vi "Test Move Vertically Outside World.vi"(8 "error in (no error)":errorcluster, 11 "Test Case In":refnum<class "World Test.lvclass">) -> (0 "error out":errorcluster, 3 "Test Case Out":refnum<class "World Test.lvclass">)   [LabVIEW 2020, in "World Test.lvclass"]
uses:
  World Test.lvclass
  C:/Program Files (x86)/National Instruments/LabVIEW 2020/vi.lib/Astemes/LUnit/Test Case.lvclass
  source/Particle/Position.ctl
  source/Particle.lvclass/Particle.ctl
  <vilib>/Astemes/LUnit/Test Case.lvclass/Test Case.ctl
  01074fa8-ee8a-411d-bc8b-fc92c4f90959.vi
  <vilib>/Astemes/LUnit/Palette/Pass.vi
  <vilib>/Astemes/LUnit/Palette/Fail.vi
  <vilib>/Astemes/LUnit/Compare Variants.vi
  <vilib>/Astemes/LUnit/Describe Comparison.vi
  <vilib>/Astemes/LUnit/Set Assertion Type.vi
  <vilib>/Astemes/LUnit/Add test result.vi
  <vilib>/Astemes/LUnit/Variant to string.vi
  <vilib>/Astemes/LUnit/LUnit Record Assertion Result.vi
  <vilib>/Astemes/LUnit/LUnit Aggregate Assertion Results.vi
  <vilib>/Astemes/LUnit/Method Result/LUnit Merge Status.vi
  <vilib>/Astemes/LUnit/LUnit Concatenate result strings.vi
  <vilib>/Utility/Data Type/Get Type Information.vi
  <vilib>/Utility/LVClass/Get LV Class Name.vi
  World Test.lvclass/World Test.ctl
  source/World/World.lvclass
  source/Particle.lvclass
panel:
  out "Position":T1
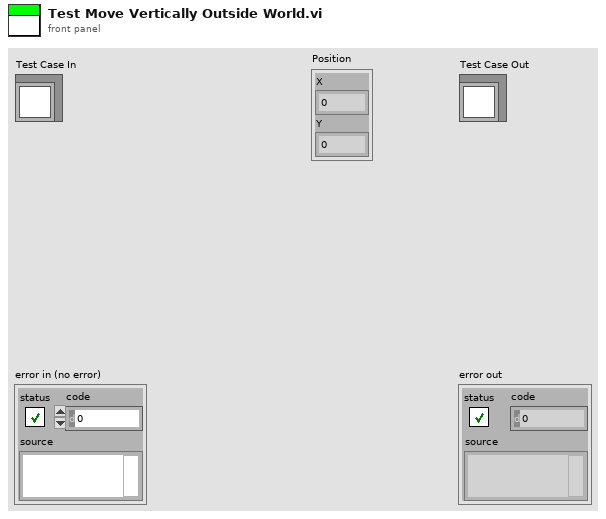
[diagram p1: front panel]
types:
  T1 = typedef "Particle.lvclass/Position.ctl" = cluster{"X":i32, "Y":i32}
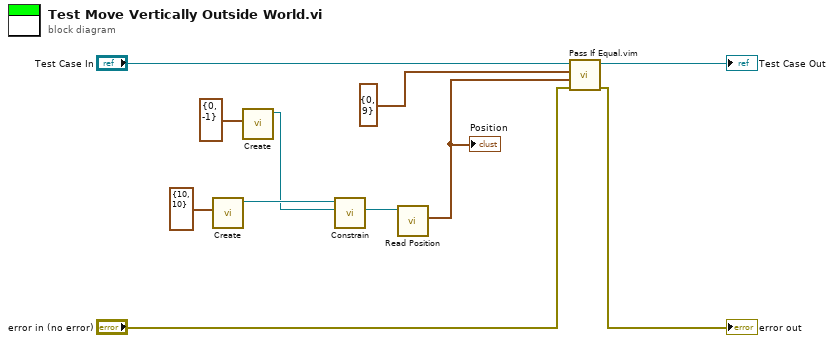
[diagram p0: block diagram]
diagram:
  n1 = call "Create.vi"("Size"=T1 {"X"=10, "Y"=10}) -> ("World out"=w5:refnum<class "World.lvclass">)  [unwired: 10 in]
  n2 = call "Create.vi"("Position"=T1 {"X"=0, "Y"=-1}) -> ("Particle out"=w4:refnum<class "Particle.lvclass">)  [unwired: 10 in]
  n3 = call "Constrain.vi"("Particle.lvclass"=w4, "World in"=w5) -> ("Particle"=w3:refnum<class "Particle.lvclass">)  [unwired: 8 in, 1 out]
  n4 = call "Read Position.vi"("Particle in"=w3) -> ("Position"=w2:T1)  [unwired: 10 in]
  "Position" <- w2
  n5 = call "Pass If Equal.vim"("error in (no error)"="error in (no error)", "Actual"=w2, "Expected"=T1 {"X"=0, "Y"=9} ("Position"), "LUnit Test Case In"="Test Case In") -> ("error out"=→"error out":errorcluster, "LUnit Test Case Out"=→"Test Case Out":refnum<class "World Test.lvclass">)  [unwired: 6 in]
